vi "切割.vi"() -> ()   [LabVIEW 2010]
uses:
  <vilib>/Instr/_visa.llb/VISA Configure Serial Port (Instr).vi
panel:
  in  "切割程序":enum32{"参数设定", "程序设定"}(tab)
  in  "baud rate":u32=9600
  in  "VISA resource name":refnum<visa-resource-name>="COM1"
  in  "data bits":u16=8 min=5 max=8 step=1
  in  "parity":u16(ring) items=["None", "Odd", "Even", "Mark", "Space"]
  in  "stop bits":u16(ring)=10 items=["1.0"=10, "1.5"=15, "2.0"=20]
  in  "flow control":u16(ring) items=["None"=0, "XON/XOFF"=1, "RTS/CTS"=2, "DTR/DSR"=4]
  in  "确认":bool
  in  "X边长（mm）":dbl
  in  "Y边长（mm）":dbl
  in  "圈数":i32
  out "滑动杆":dbl(slide) scale=0.0..100.0
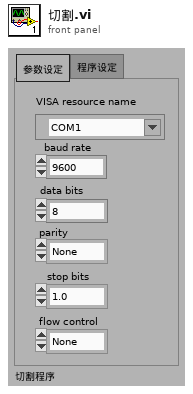
[diagram p1: front panel]
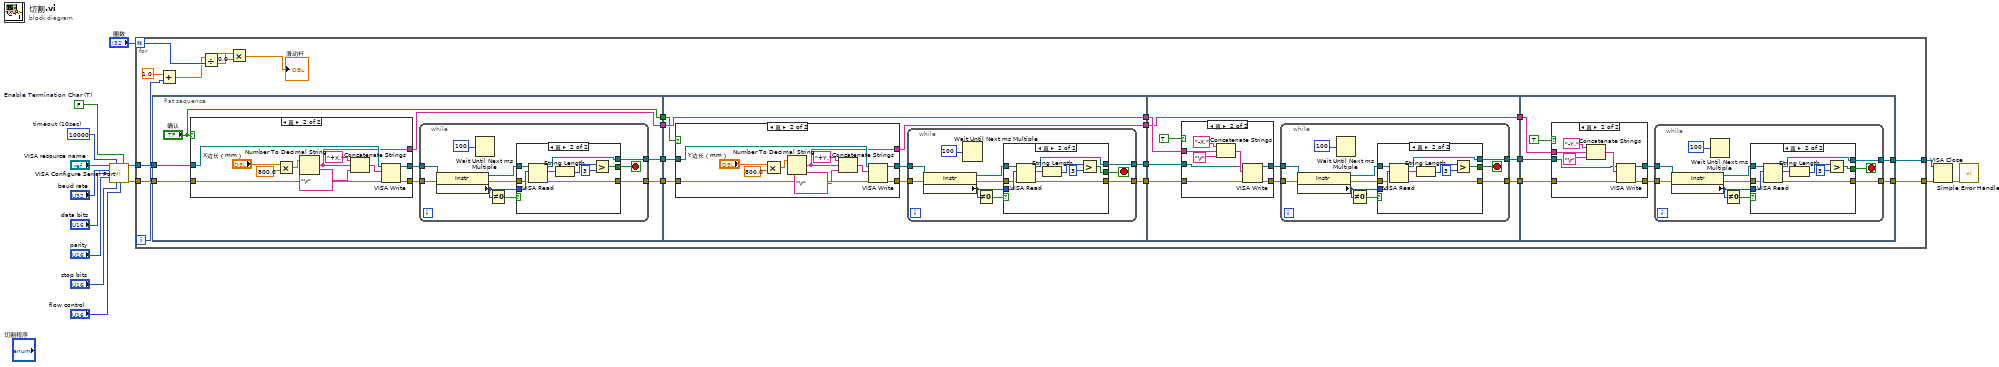
[diagram p0: block diagram]
diagram:
  w10 = FALSE  # Enable Termination Char (T)
  w11 = u32 10000  # timeout (10sec)
  n1 = call-poly "VISA Configure Serial Port"("VISA resource name"="VISA resource name", "timeout (10sec)"=w11, "Enable Termination\nChar (T)"=w10, "baud rate (9600)"="baud rate", "data bits (8)"="data bits", "parity (0:none)"="parity", "stop bits (10: 1 bit)"="stop bits", "flow control (0:none)"="flow control") -> ("VISA resource name out"=w6:refnum<visa-resource-name>, "error out"=w5:errorcluster)  [unwired: 1 in, 5 out]
  n2 = for {
    N: "圈数" -> [w21]
    tunnel: w6 -> [w36]
    tunnel: w5 -> [w33]
    tunnel: [w23] -> w3
    tunnel: [w22] -> w2
    i -> [w16]
    n3 = flat-sequence {
      tunnel: w36 -> [w42]
      tunnel: [w41] -> w35
      tunnel: [w40] -> w34
      tunnel: w33 -> [w39]
      tunnel: [w38] -> w29
      tunnel: ["确认"] -> w24
      tunnel: w35 -> [w81]
      tunnel: w34 -> [w80]
      tunnel: [w79] -> w32
      tunnel: [w78] -> w31
      tunnel: [w77] -> w30
      tunnel: w29 -> [w77]
      tunnel: [w76] -> w25
      tunnel: w24 -> [w75]
      tunnel: w32 -> [w120]
      tunnel: w31 -> [w119]
      tunnel: w30 -> [w118]
      tunnel: [w117] -> w28
      tunnel: [w116] -> w27
      tunnel: [w115] -> w26
      tunnel: w25 -> [w115]
      tunnel: w28 -> [w155]
      tunnel: w27 -> [w154]
      tunnel: w26 -> [w153]
      tunnel: [w151] -> w23
      tunnel: [w150] -> w22
      frame #0 {
        n4 = case shown="真" "确认" {
          tunnel: [_ w74] -> w43
          tunnel: [_ w73] -> w44
          tunnel: w42 -> [_ w72]
          tunnel: w39 -> [_ w66]
          tunnel: [_ w65] -> w38
          frame False {
          }
          frame True {
            n5 = Multiply(x="X边长（mm）", y=800.0) -> (x*y=w69:dbl)
            n6 = Number To Decimal String(number=w69) -> (decimal integer string=w65:string)  [unwired: 1 out]
            n7 = Concatenate Strings("+X," ("字符串"), w65, "\r" ("字符串")) -> (w67:string)
            n8 = VISA Write(VISA resource name=w72, write buffer=w67, error in (no error)=w66) -> (VISA resource name out=w73:refnum<visa-resource-name>, error out=w74:errorcluster)  [unwired: 1 out]
          }
        }
        n9 = while {
          tunnel: w44 -> [w53]
          tunnel: w43 -> [w52]
          tunnel: [w47] -> w41
          tunnel: [w46] -> w40
          stop <- w45 stop-if-true
          n10 = property class="Instr"(reference=w53, error in=w52) -> (reference out=w54:refnum<visa-resource-name>, error out=w51:errorcluster, "Serial Settings:Number of Bytes at Serial Port"=w49:u32)
          n11 = Wait Until Next ms Multiple(millisecond multiple=u32 100 ("毫秒倍数")) -> ()  [unwired: 1 out]
          n12 = Not Equal To 0?(x=w49) -> (x != 0?=w48:bool)
          n13 = case shown="真" w48 {
            tunnel: w54 -> [_ w63]
            tunnel: w49 -> [_ w62]
            tunnel: w51 -> [_ w61]
            tunnel: [_ w60] -> w47
            tunnel: [_ w59] -> w46
            tunnel: [_ w55] -> w45
            frame False {
            }
            frame True {
              n14 = VISA Read(VISA resource name=w63, byte count=w62, error in (no error)=w61) -> (VISA resource name out=w60:refnum<visa-resource-name>, read buffer=w58:string, error out=w59:errorcluster)  [unwired: 1 out]
              n15 = String Length(string=w58) -> (length=w57:i32)
              n16 = Greater?(x=w57, y=3) -> (0:w55:bool)
            }
          }
        }
      }
      frame #1 {
        n17 = case shown="真" w75 {
          tunnel: [_ w94] -> w82
          tunnel: [_ w93] -> w83
          tunnel: w81 -> [_ w87]
          tunnel: w80 -> [_ w86]
          tunnel: [_ w85] -> w76
          frame False {
          }
          frame True {
            n18 = Multiply(x="Y边长（mm）", y=800.0) -> (x*y=w90:dbl)
            n19 = Number To Decimal String(number=w90) -> (decimal integer string=w85:string)  [unwired: 1 out]
            n20 = Concatenate Strings("+Y," ("字符串"), w85, "\r" ("字符串")) -> (w88:string)
            n21 = VISA Write(VISA resource name=w87, write buffer=w88, error in (no error)=w86) -> (VISA resource name out=w93:refnum<visa-resource-name>, error out=w94:errorcluster)  [unwired: 1 out]
          }
        }
        n22 = while {
          tunnel: [w99] -> w79
          tunnel: [w98] -> w78
          tunnel: w83 -> [w97]
          tunnel: w82 -> [w96]
          stop <- w95 stop-if-true
          n23 = property class="Instr"(reference=w97, error in=w96) -> (reference out=w104:refnum<visa-resource-name>, error out=w103:errorcluster, "Serial Settings:Number of Bytes at Serial Port"=w101:u32)
          n24 = Wait Until Next ms Multiple(millisecond multiple=u32 100 ("毫秒倍数")) -> ()  [unwired: 1 out]
          n25 = Not Equal To 0?(x=w101) -> (x != 0?=w100:bool)
          n26 = case shown="真" w100 {
            tunnel: w104 -> [_ w113]
            tunnel: w101 -> [_ w112]
            tunnel: w103 -> [_ w111]
            tunnel: [_ w110] -> w99
            tunnel: [_ w109] -> w98
            tunnel: [_ w105] -> w95
            frame False {
            }
            frame True {
              n27 = VISA Read(VISA resource name=w113, byte count=w112, error in (no error)=w111) -> (VISA resource name out=w110:refnum<visa-resource-name>, read buffer=w108:string, error out=w109:errorcluster)  [unwired: 1 out]
              n28 = String Length(string=w108) -> (length=w106:i32)
              n29 = Greater?(x=w106, y=3) -> (0:w105:bool)
            }
          }
        }
      }
      frame #2 {
        n30 = case shown="真" TRUE {
          tunnel: [_ w130] -> w121
          tunnel: [_ w129] -> w122
          tunnel: w120 -> [_ w125]
          tunnel: w119 -> [_ w124]
          tunnel: w118 -> [_ w123]
          frame False {
          }
          frame True {
            n31 = Concatenate Strings("-X," ("字符串"), w123, "\r" ("字符串")) -> (w126:string)
            n32 = VISA Write(VISA resource name=w125, write buffer=w126, error in (no error)=w124) -> (VISA resource name out=w129:refnum<visa-resource-name>, error out=w130:errorcluster)  [unwired: 1 out]
          }
        }
        n33 = while {
          tunnel: [w135] -> w117
          tunnel: [w134] -> w116
          tunnel: w122 -> [w133]
          tunnel: w121 -> [w132]
          stop <- w131 stop-if-true
          n34 = property class="Instr"(reference=w133, error in=w132) -> (reference out=w140:refnum<visa-resource-name>, error out=w139:errorcluster, "Serial Settings:Number of Bytes at Serial Port"=w137:u32)
          n35 = Wait Until Next ms Multiple(millisecond multiple=u32 100 ("毫秒倍数")) -> ()  [unwired: 1 out]
          n36 = Not Equal To 0?(x=w137) -> (x != 0?=w136:bool)
          n37 = case shown="真" w136 {
            tunnel: w140 -> [_ w149]
            tunnel: w137 -> [_ w148]
            tunnel: w139 -> [_ w147]
            tunnel: [_ w146] -> w135
            tunnel: [_ w145] -> w134
            tunnel: [_ w141] -> w131
            frame False {
            }
            frame True {
              n38 = VISA Read(VISA resource name=w149, byte count=w148, error in (no error)=w147) -> (VISA resource name out=w146:refnum<visa-resource-name>, read buffer=w144:string, error out=w145:errorcluster)  [unwired: 1 out]
              n39 = String Length(string=w144) -> (length=w142:i32)
              n40 = Greater?(x=w142, y=3) -> (0:w141:bool)
            }
          }
        }
      }
      frame #3 {
        n41 = case shown="真" TRUE {
          tunnel: [_ w165] -> w156
          tunnel: [_ w164] -> w157
          tunnel: w155 -> [_ w160]
          tunnel: w154 -> [_ w159]
          tunnel: w153 -> [_ w158]
          frame False {
          }
          frame True {
            n42 = Concatenate Strings("-Y," ("字符串"), w158, "\r" ("字符串")) -> (w161:string)
            n43 = VISA Write(VISA resource name=w160, write buffer=w161, error in (no error)=w159) -> (VISA resource name out=w164:refnum<visa-resource-name>, error out=w165:errorcluster)  [unwired: 1 out]
          }
        }
        n44 = while {
          tunnel: [w170] -> w151
          tunnel: [w169] -> w150
          tunnel: w157 -> [w168]
          tunnel: w156 -> [w167]
          stop <- w166 stop-if-true
          n45 = property class="Instr"(reference=w168, error in=w167) -> (reference out=w175:refnum<visa-resource-name>, error out=w174:errorcluster, "Serial Settings:Number of Bytes at Serial Port"=w172:u32)
          n46 = Wait Until Next ms Multiple(millisecond multiple=u32 100 ("毫秒倍数")) -> ()  [unwired: 1 out]
          n47 = Not Equal To 0?(x=w172) -> (x != 0?=w171:bool)
          n48 = case shown="真" w171 {
            tunnel: w175 -> [_ w184]
            tunnel: w172 -> [_ w183]
            tunnel: w174 -> [_ w182]
            tunnel: [_ w181] -> w170
            tunnel: [_ w180] -> w169
            tunnel: [_ w176] -> w166
            frame False {
            }
            frame True {
              n49 = VISA Read(VISA resource name=w184, byte count=w183, error in (no error)=w182) -> (VISA resource name out=w181:refnum<visa-resource-name>, read buffer=w179:string, error out=w180:errorcluster)  [unwired: 1 out]
              n50 = String Length(string=w179) -> (length=w177:i32)
              n51 = Greater?(x=w177, y=3) -> (0:w176:bool)
            }
          }
        }
      }
    }
    n52 = Add(x=1.0, y=w16) -> (x+y=w15:dbl)
    n53 = Divide(x=w15, y=w21) -> (x/y=w20:dbl)
    n54 = Multiply(x=w20, y=100.0) -> (x*y=→"滑动杆":dbl)
  }
  n55 = VISA Close(VISA resource name=w3, error in (no error)=w2) -> (error out=w4:errorcluster)
  n56 = call <vilib>:"Simple Error Handler.vi"("error in (no error)"=w4) -> ()  [unwired: 1 in, 8 out]
